vi "Set_Tab_Pages.vi"(7 "Pages visible? (false)":bool, 8 "Status/Errors in":refnum<vi>, 9 "Control Parameters [] in":T15[](array[typedef]) {"Aux Byte Value" format="%02x"; "Max Real Value" format="%#_6e"; "Min Real Value" format="%#_6e"; "dReal/dByte" format="%#_6e"; "Byte Value" format="%02x"; "Identifier" format="%02x"}, 10 "Main parameters in":T1={"Mode"={"Mode"=enum."Dialog", "Expert?"=FALSE, "Dialog?"=FALSE}, "Stop loop"={"Settings changed?"=FALSE, "Stop?"=refnum}, "Send message"={"Send mode"=enum."Get parameters", "Set parameter list"=0, "Get parameter list"=0, "Reset device"=0, "Length set settings message"=0, "Reset buttons?"=FALSE, "Reset Master?"=enum."General"}, "Write settings"={"Options"=enum."File 1"}, "Settings state"={"MAS locked?"=refnum, "SLV locked?"=refnum}, "Button refs"={"Stop program"=refnum, "Save settings"=refnum, "DAQ mode"=refnum, "Reset settings"=refnum, "Apply settings"=refnum, "Reset MAS"=refnum, "Reset SLV"=refnum, "Local DBase?"=refnum, "Last value DBase"=FALSE, "Database"=refnum, "Calibration"=refnum, "Save settings 2"=refnum}, "Update screen"={"Detector number"=0, "Hardware"=enum."None"}, "Files"={"Path config file"=path "", "Path def. ini file"=path "", "Path ini file 1"=path "", "Path ini file 2"=path "", "Path RBF file"=path ""}, "DB connection"={"connection reference"=refnum, "Connected?"=refnum, "ODBC Name"=""}, "Status_id"=refnum, "Time difference"=refnum, "Satellites"=refnum, "Alignment parameters"=refnum, "Page Statistics 2"=refnum, "Database"=refnum, "Page Statistics"=refnum} {"Update screen"."Detector number" format="%#.0f"; "Send message"."Reset device" format="%x"; "Send message"."Get parameter list" format="%x"; "Send message"."Set parameter list" format="%x"}, 11 "Device in":refnum<vi>) -> (0 "Status/Errors out":refnum<vi>, 1 "Control Parameters [] out":T15[](array[typedef]) {"Aux Byte Value" format="%02x"; "Max Real Value" format="%#_6e"; "Min Real Value" format="%#_6e"; "dReal/dByte" format="%#_6e"; "Byte Value" format="%02x"; "Identifier" format="%02x"}, 2 "Main parameters out":T1={"Mode"={"Mode"=enum."Dialog", "Expert?"=FALSE, "Dialog?"=FALSE}, "Stop loop"={"Settings changed?"=FALSE, "Stop?"=refnum}, "Send message"={"Send mode"=enum."Get parameters", "Set parameter list"=0, "Get parameter list"=0, "Reset device"=0, "Length set settings message"=0, "Reset buttons?"=FALSE, "Reset Master?"=enum."General"}, "Write settings"={"Options"=enum."File 1"}, "Settings state"={"MAS locked?"=refnum, "SLV locked?"=refnum}, "Button refs"={"Stop program"=refnum, "Save settings"=refnum, "DAQ mode"=refnum, "Reset settings"=refnum, "Apply settings"=refnum, "Reset MAS"=refnum, "Reset SLV"=refnum, "Local DBase?"=refnum, "Last value DBase"=FALSE, "Database"=refnum, "Calibration"=refnum, "Save settings 2"=refnum}, "Update screen"={"Detector number"=0, "Hardware"=enum."None"}, "Files"={"Path config file"=path "", "Path def. ini file"=path "", "Path ini file 1"=path "", "Path ini file 2"=path "", "Path RBF file"=path ""}, "DB connection"={"connection reference"=refnum, "Connected?"=refnum, "ODBC Name"=""}, "Status_id"=refnum, "Time difference"=refnum, "Satellites"=refnum, "Alignment parameters"=refnum, "Page Statistics 2"=refnum, "Database"=refnum, "Page Statistics"=refnum} {"Update screen"."Detector number" format="%#.0f"; "Send message"."Reset device" format="%x"; "Send message"."Get parameter list" format="%x"; "Send message"."Set parameter list" format="%x"}, 3 "Device out":refnum<vi>)   [LabVIEW 2010]
uses:
  Controls/Control_Parameters.ctl
  Controls/Master.ctl
  Controls/Main_Parameters.ctl
  Controls/Mode.ctl
  Controls/Stop_Loop.ctl
  Controls/Send_Message.ctl
  Controls/Send_Message_Mode.ctl
  Controls/Write_Settings.ctl
  Controls/Write_Settings_Options.ctl
  Controls/Settings_State.ctl
  Controls/Button_Refs.ctl
  Controls/Update_Screen.ctl
  Controls/Files.ctl
  Controls/DB_Connection.ctl
  database/Connection.llb/Conn ObjectReference.ctl
  Controls/Device_Elements.ctl
  Controls/Get_Set_Device_Options.ctl
  Controls/Get_Set_Buttons_mode.ctl
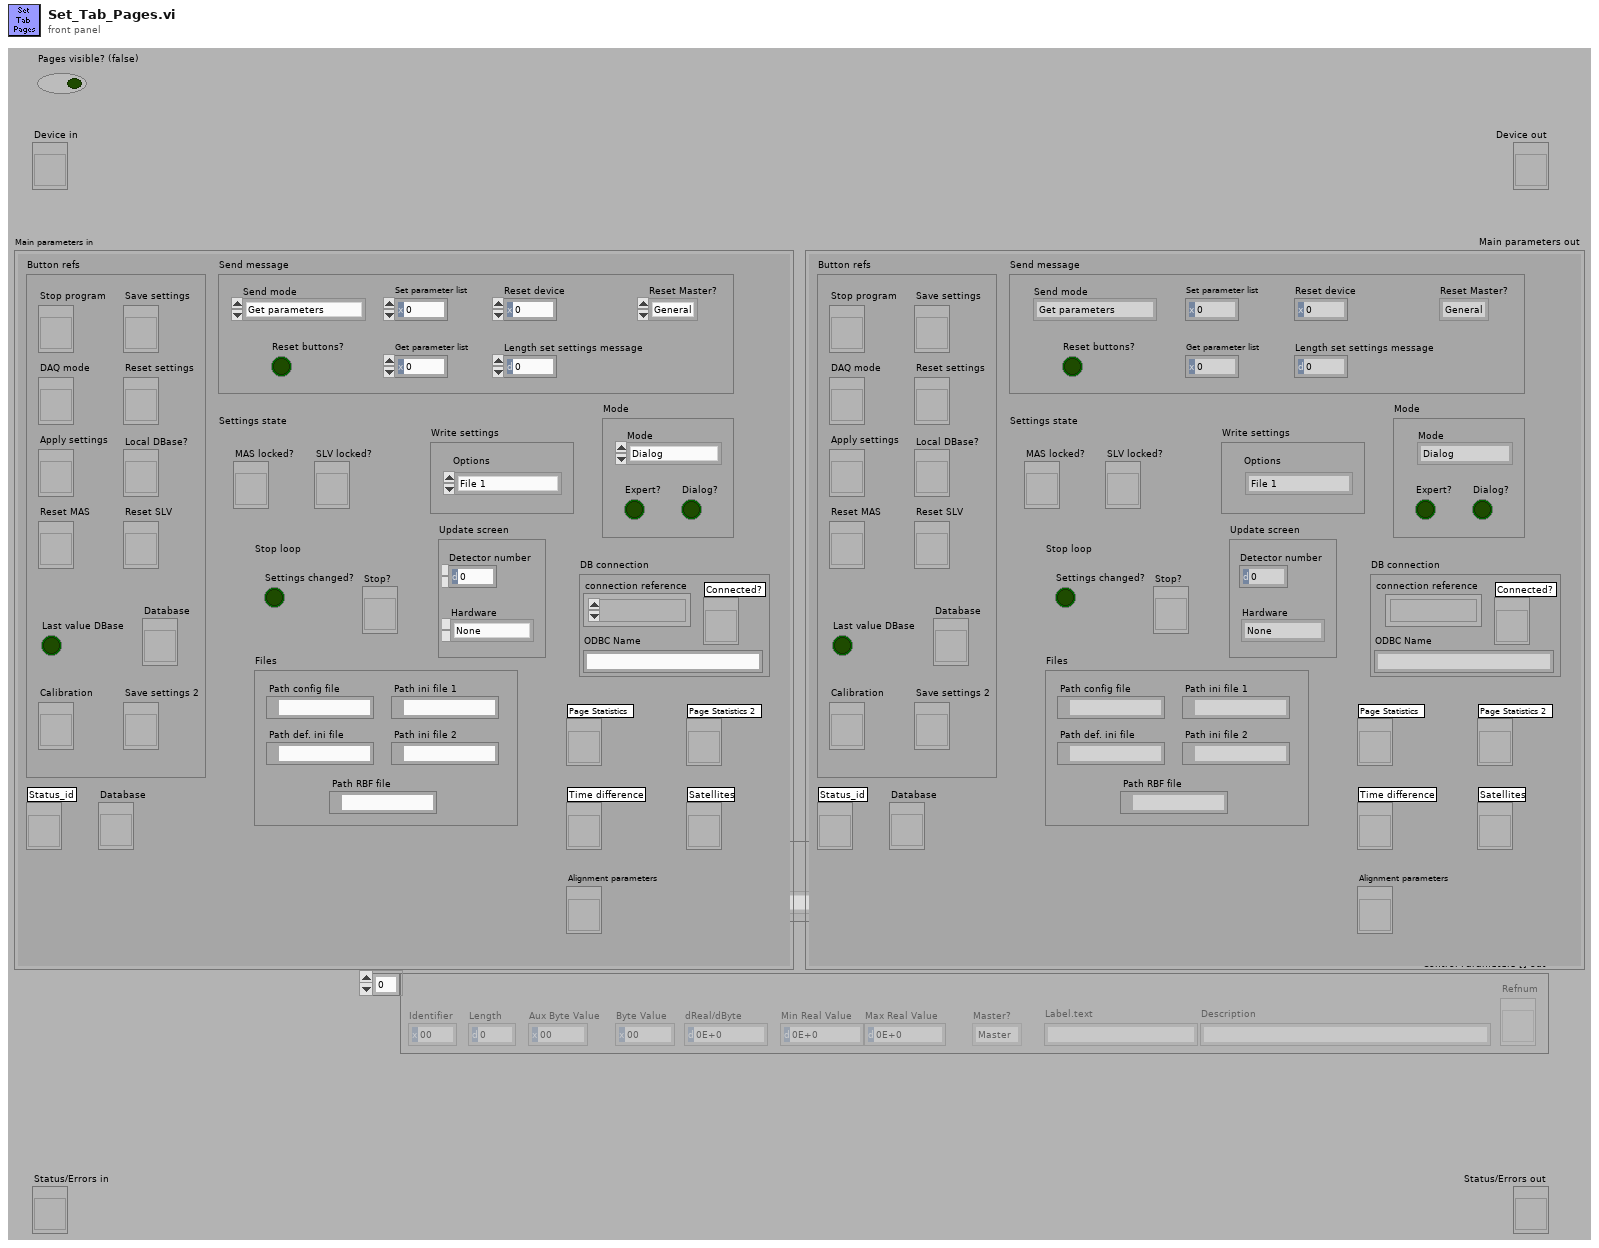
[diagram p1: front panel]
types:
  T1 = typedef "Main_Parameters.ctl" = cluster{"Mode":T2, "Stop loop":T3, "Send message":T4, "Write settings":T7, "Settings state":T9, "Button refs":T10, "Update screen":T11, "Files":T12, "DB connection":T13, "Status_id":refnum<vi>, "Time difference":refnum<vi>, "Satellites":refnum<vi>, "Alignment parameters":refnum<vi>, "Page Statistics 2":refnum<vi>, "Database":refnum<vi>, "Page Statistics":refnum<vi>}
  T2 = typedef "Mode.ctl" = cluster{"Mode":enum8{"Stop", "Dialog", "Hisparc II", "Hisparc II DAQ", "Alignment"}, "Expert?":bool, "Dialog?":bool}
  T3 = typedef "Stop_Loop.ctl" = cluster{"Settings changed?":bool, "Stop?":refnum<vi>}
  T4 = typedef "Send_Message.ctl" = cluster{"Send mode":T5, "Set parameter list":u8, "Get parameter list":u8, "Reset device":u8, "Length set settings message":i32, "Reset buttons?":bool, "Reset Master?":T6}
  T5 = typedef "Send_Message_Mode.ctl" = enum16{"Get parameters", "Set parameters", "From front panel", "From parameters", "Reset device", "Alignment"}
  T6 = typedef "Master.ctl" = enum16{"Master", "Slave", "General"}
  T7 = typedef "Write_Settings.ctl" = cluster{"Options":T8}
  T8 = typedef "Write_Settings_Options.ctl" = enum16{"File 1", "File 2", "Alignment", "Reset"}
  T9 = typedef "Settings_State.ctl" = cluster{"MAS locked?":refnum<vi>, "SLV locked?":refnum<vi>}
  T10 = typedef "Button_Refs.ctl" = cluster{"Stop program":refnum<vi>, "Save settings":refnum<vi>, "DAQ mode":refnum<vi>, "Reset settings":refnum<vi>, "Apply settings":refnum<vi>, "Reset MAS":refnum<vi>, "Reset SLV":refnum<vi>, "Local DBase?":refnum<vi>, "Last value DBase":bool, "Database":refnum<vi>, "Calibration":refnum<vi>, "Save settings 2":refnum<vi>}
  T11 = typedef "Update_Screen.ctl" = cluster{"Detector number":u16, "Hardware":enum8{"None", "HiSPARC I", "HiSPARC II", "HiSPARC III", "Unknown"}}
  T12 = typedef "Files.ctl" = cluster{"Path config file":path, "Path def. ini file":path, "Path ini file 1":path, "Path ini file 2":path, "Path RBF file":path}
  T13 = typedef "DB_Connection.ctl" = cluster{"connection reference":T14, "Connected?":refnum<vi>, "ODBC Name":string}
  T14 = typedef "Conn ObjectReference.ctl" = refnum<k1>
  T15 = typedef "Control_Parameters.ctl" = cluster{"Identifier":u8, "Length":u16, "Byte Value":u32, "dReal/dByte":dbl, "Min Real Value":dbl, "Max Real Value":dbl, "Master?":T6, "Label.text":string, "Description":string, "Refnum":refnum<vi>, "Aux Byte Value":u32}
  T16 = typedef "Get_Set_Device_Options.ctl" = enum16{"Get", "Get cluster", "Set"}
  T17 = typedef "Device_Elements.ctl" = enum16{"Default", "Master?", "Connected?", "Status", "Disconnect?", "Handle", "Version number"}
  T18 = enum8{"Stop", "Dialog", "Hisparc II", "Hisparc II DAQ", "Alignment"}
  T19 = typedef "Get_Set_Buttons_mode.ctl" = enum16{"Get", "Get DAQ", "Set", "Set settings"}
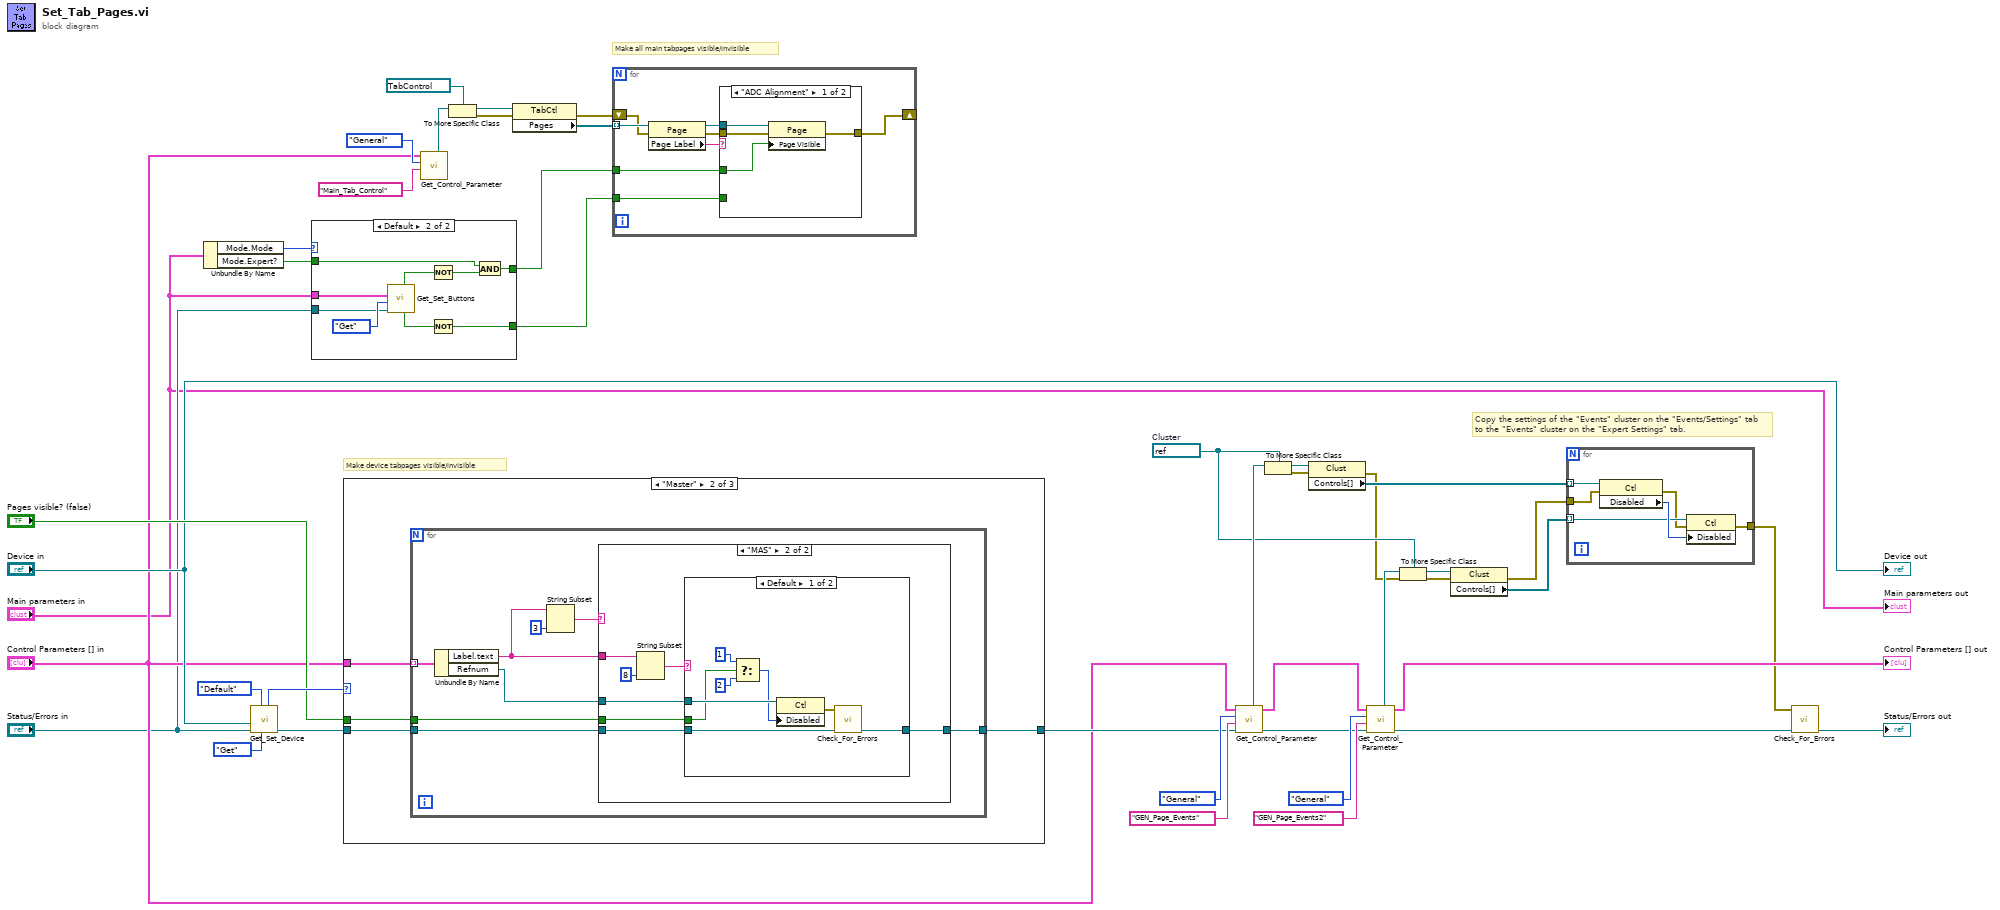
[diagram p0: block diagram]
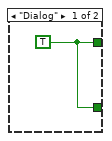
[diagram p2: hidden frame]
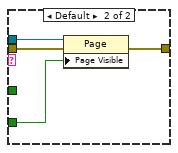
[diagram p3: hidden frame]
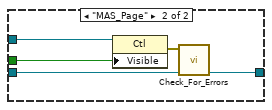
[diagram p6: hidden frame]
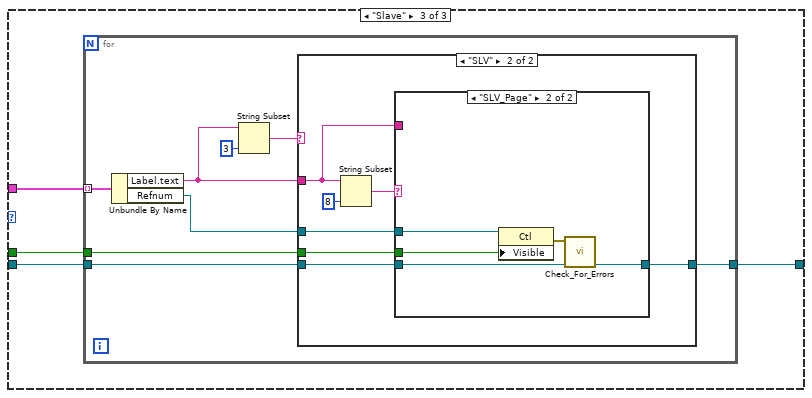
[diagram p7: hidden frame]
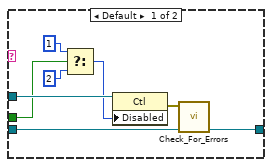
[diagram p9: hidden frame]
diagram:
  w25 = refnum<vi> refnum  # Cluster
  # "Make all main tabpages visible/invisible"
  # "Copy the settings of the \"Events\" cluster on the \"Events/Settings\" tab\nto the \"Events\" cluster on the \"Expert Settings\" tab."
  # "Make device tabpages visible/invisible"
  n1 = Unbundle By Name("Main parameters in") -> ("Mode.Mode"=w2:T18, "Mode.Expert?"=w3:bool)
  n2 = call "Get_Set_Device.vi"("Get/Set"=Get_Set_Device_Options."Get", "Element"=Device_Elements."Default", "Status/Errors in"="Status/Errors in", "Device in"="Device in") -> ("Status/Errors out"=w21:refnum<vi>, "Master?"=w20:T6)  [unwired: 1 in, 5 out]
  n3 = case shown="Default" w2 {
    tunnel: [w44 w52] -> w7
    tunnel: [w44 w48] -> w6
    tunnel: "Main parameters in" -> [_ w46]
    tunnel: "Status/Errors in" -> [_ w47]
    tunnel: w3 -> [_ w45]
    frame "Dialog" {
      w44 = TRUE
    }
    frame Default {
      n4 = call "Get_Set_Buttons.vi"("Status/Errors in"=w47, "Set?"=Get_Set_Buttons_mode."Get", "Main parameters"=w46) -> ("Calibration value"=w51:bool, "DAQ mode value"=w50:bool)  [unwired: 1 in, 6 out]
      n5 = Not(x=w50) -> (.not. x?=w49:bool)
      n6 = Not(x=w51) -> (.not. x?=w52:bool)
      n7 = And(x=w45, y=w49) -> (x .and. y?=w48:bool)
    }
  }
  n8 = case shown="\"Master\"" w20 {
    tunnel: w21 -> [w54 w57 w91]
    tunnel: [w54 w55 w89] -> w37
    tunnel: "Control Parameters [] in" -> [_ w58 w90]
    tunnel: "Pages visible? (false)" -> [_ w56 w88]
    frame Default {
    }
    frame "Master" {
      n9 = for {
        tunnel: w58 -> [w66] mode=indexing
        tunnel: w57 -> [w65]
        tunnel: [w64] -> w55
        tunnel: w56 -> [w62]
        n10 = Unbundle By Name(w66) -> ("Label.text"=w59:string, "Refnum"=w63:refnum<vi>)
        n11 = String Subset(string=w59, length (rest)=3 ("length (rest)")) -> (substring=w60:string)  [unwired: 1 out]
        n12 = case shown="\"MAS\"" w60 {
          tunnel: w65 -> [w67 w74]
          tunnel: [w67 w73] -> w64
          tunnel: w63 -> [_ w72]
          tunnel: w62 -> [_ w71]
          tunnel: w59 -> [_ w68]
          frame Default {
          }
          frame "MAS" {
            n13 = String Subset(string=w68, length (rest)=8 ("length (rest)")) -> (substring=w69:string)  [unwired: 1 out]
            n14 = case shown="Default" w69 {
              tunnel: w72 -> [w79 w84]
              tunnel: w74 -> [w81 w86]
              tunnel: [w80 w83] -> w73
              tunnel: w71 -> [w78 w85]
              frame Default {
                n15 = Select(t=u8 1 ("Disabled"), s=w78, f=u8 2) -> (s? t:f=w75:u8)
                n16 = property class="Ctl"(reference=w79, "Disabled"=w75) -> (error out=w82:errorcluster)  [unwired: 1 in, 1 out]
                n17 = call "Check_For_Errors.vi"("Status/Errors in"=w81, "error in"=w82) -> ("Status/Errors out"=w80:refnum<vi>)  [unwired: 9 out]
              }
              frame "MAS_Page" {
                n18 = property class="Ctl"(reference=w84, "Visible"=w85) -> (error out=w87:errorcluster)  [unwired: 1 in, 1 out]
                n19 = call "Check_For_Errors.vi"("Status/Errors in"=w86, "error in"=w87) -> ("Status/Errors out"=w83:refnum<vi>)  [unwired: 9 out]
              }
            }
          }
        }
      }
    }
    frame "Slave" {
      n20 = for {
        tunnel: w90 -> [w99] mode=indexing
        tunnel: w91 -> [w98]
        tunnel: [w97] -> w89
        tunnel: w88 -> [w95]
        n21 = Unbundle By Name(w99) -> ("Label.text"=w92:string, "Refnum"=w96:refnum<vi>)
        n22 = String Subset(string=w92, length (rest)=3 ("length (rest)")) -> (substring=w93:string)  [unwired: 1 out]
        n23 = case shown="\"SLV\"" w93 {
          tunnel: w98 -> [w100 w107]
          tunnel: [w100 w106] -> w97
          tunnel: w96 -> [_ w105]
          tunnel: w95 -> [_ w104]
          tunnel: w92 -> [_ w101]
          frame Default {
          }
          frame "SLV" {
            n24 = String Subset(string=w101, length (rest)=8 ("length (rest)")) -> (substring=w102:string)  [unwired: 1 out]
            n25 = case shown="\"SLV_Page\"" w102 {
              tunnel: w105 -> [w112 w119]
              tunnel: w107 -> [w114 w117]
              tunnel: [w113 w116] -> w106
              tunnel: w101 -> [_ _]
              tunnel: w104 -> [w111 w118]
              frame Default {
                n26 = Select(t=u8 1 ("Disabled"), s=w111, f=u8 2) -> (s? t:f=w108:u8)
                n27 = property class="Ctl"(reference=w112, "Disabled"=w108) -> (error out=w115:errorcluster)  [unwired: 1 in, 1 out]
                n28 = call "Check_For_Errors.vi"("Status/Errors in"=w114, "error in"=w115) -> ("Status/Errors out"=w113:refnum<vi>)  [unwired: 9 out]
              }
              frame "SLV_Page" {
                n29 = property class="Ctl"(reference=w119, "Visible"=w118) -> (error out=w120:errorcluster)  [unwired: 1 in, 1 out]
                n30 = call "Check_For_Errors.vi"("Status/Errors in"=w117, "error in"=w120) -> ("Status/Errors out"=w116:refnum<vi>)  [unwired: 9 out]
              }
            }
          }
        }
      }
    }
  }
  n31 = call "Get_Control_Parameter.vi"("Label.text in"="Main_Tab_Control", "Master?"=Master."General", "Control Parameters [] in"="Control Parameters [] in") -> ("Refnum"=w10:refnum<vi>)  [unwired: 1 in, 7 out]
  n32 = To More Specific Class(target class=refnum<vi> refnum ("Main Tab Control in"), reference=w10) -> (specific class reference=w8:refnum<vi>, error out=w9:errorcluster)  [unwired: 1 in]
  n33 = property class="TabCtl"(reference=w8, error in=w9) -> (error out=w14:errorcluster, "Pages"=w15:refnum<vi>[])  [unwired: 1 out]
  n34 = for {
    tunnel: w15 -> [w128] mode=indexing
    shift-right: [w123] -> _
    shift-left: w14 -> [w125]
    tunnel: w6 -> [w122]
    tunnel: w7 -> [w121]
    n35 = property class="Page"(reference=w128, error in=w125) -> (reference out=w126:refnum<vi>, error out=w124:errorcluster, "Page Label"=w127:string)
    n36 = case shown="\"ADC Alignment\"" w127 {
      tunnel: w126 -> [w132 w136]
      tunnel: w124 -> [w131 w135]
      tunnel: [w130 w134] -> w123
      tunnel: w122 -> [w129 _]
      tunnel: w121 -> [_ w133]
      frame "ADC Alignment" {
        n37 = property class="Page"(reference=w132, error in=w131, "Page Visible"=w129) -> (error out=w130:errorcluster)  [unwired: 1 out]
      }
      frame Default {
        n38 = property class="Page"(reference=w136, error in=w135, "Page Visible"=w133) -> (error out=w134:errorcluster)  [unwired: 1 out]
      }
    }
  }
  n39 = call "Get_Control_Parameter.vi"("Status/Errors in"=w37, "Label.text in"="GEN_Page_Events", "Master?"=Master."General", "Control Parameters [] in"="Control Parameters [] in") -> ("Status/Errors out"=w28:refnum<vi>, "Control Parameters [] out"=w38:T15[], "Refnum"=w34:refnum<vi>)  [unwired: 5 out]
  n40 = To More Specific Class(target class=w25, reference=w34) -> (specific class reference=w33:refnum<vi>, error out=w27:errorcluster)  [unwired: 1 in]
  n41 = property class="Clust"(reference=w33, error in=w27) -> (error out=w24:errorcluster, "Controls[]"=w32:refnum<vi>[])  [unwired: 1 out]
  n42 = call "Get_Control_Parameter.vi"("Status/Errors in"=w28, "Label.text in"="GEN_Page_Events2", "Master?"=Master."General", "Control Parameters [] in"=w38) -> ("Status/Errors out"=w39:refnum<vi>, "Control Parameters [] out"=→"Control Parameters [] out":T15[], "Refnum"=w30:refnum<vi>)  [unwired: 5 out]
  n43 = To More Specific Class(target class=w25, reference=w30, error in=w24) -> (specific class reference=w31:refnum<vi>, error out=w26:errorcluster)
  n44 = property class="Clust"(reference=w31, error in=w26) -> (error out=w23:errorcluster, "Controls[]"=w29:refnum<vi>[])  [unwired: 1 out]
  n45 = for {
    tunnel: w32 -> [w142] mode=indexing
    tunnel: w29 -> [w140] mode=indexing
    tunnel: [w138] -> w22
    tunnel: w23 -> [w137]
    n46 = property class="Ctl"(reference=w142, error in=w137) -> (error out=w139:errorcluster, "Disabled"=w141:u8)  [unwired: 1 out]
    n47 = property class="Ctl"(reference=w140, error in=w139, "Disabled"=w141) -> (error out=w138:errorcluster)  [unwired: 1 out]
  }
  n48 = call "Check_For_Errors.vi"("Status/Errors in"=w39, "error in"=w22) -> ("Status/Errors out"=→"Status/Errors out":refnum<vi>)  [unwired: 9 out]
  "Device out" <- "Device in"
  "Main parameters out" <- "Main parameters in"
